vi "GVSDataView Mark Frame Below.vi"() -> ()   [LabVIEW 2013]
uses:
  <vilib>/Utility/miscctls.llb/LVPositionTypeDef.ctl
  SubVI/GVSMain Sub Window Global.vi
  GVSNew View Global.vi
panel:
  in  "sMe":string
  in  "bShow":bool=TRUE
  in  "Below":bool
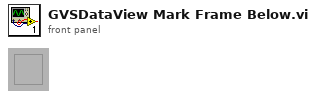
[diagram p1: front panel]
types:
  T1 = typedef "LVPositionTypeDef.ctl" = cluster{"Left":i32, "Top":i32}
  T2 = typedef "LVRectTypeDef.ctl" = cluster{"Left":i16, "Top":i16, "Right":i16, "Bottom":i16}
  T3 = typedef "Graph Main Info Cluster.ctl" = cluster{"Selected_BarIdx":i32, "Selected_PanelIdx":i32, "Graph Main VIRef":refnum<vi>, "ToolBarClick":bool, "Spliter Ref Array":refnum<vi>[], "Panel Ref Array":refnum<vi>[], "Spliter_matrix":i32[][], "Panel_matrix":i32[][], "child_spliterIdx_matrix":i32[][], "split_pos_matrix":i32[][], "Title State":bool, "sQueueName":string, "Frame nID":i32, "Graph VIRef Array":cluster{"Graph VIRef":refnum<vi>, "Panel Idx":i32, "Frame VIRef":refnum<vi>, "Icon Ring":i32, "Graph Type":string}[], "View Type":string}
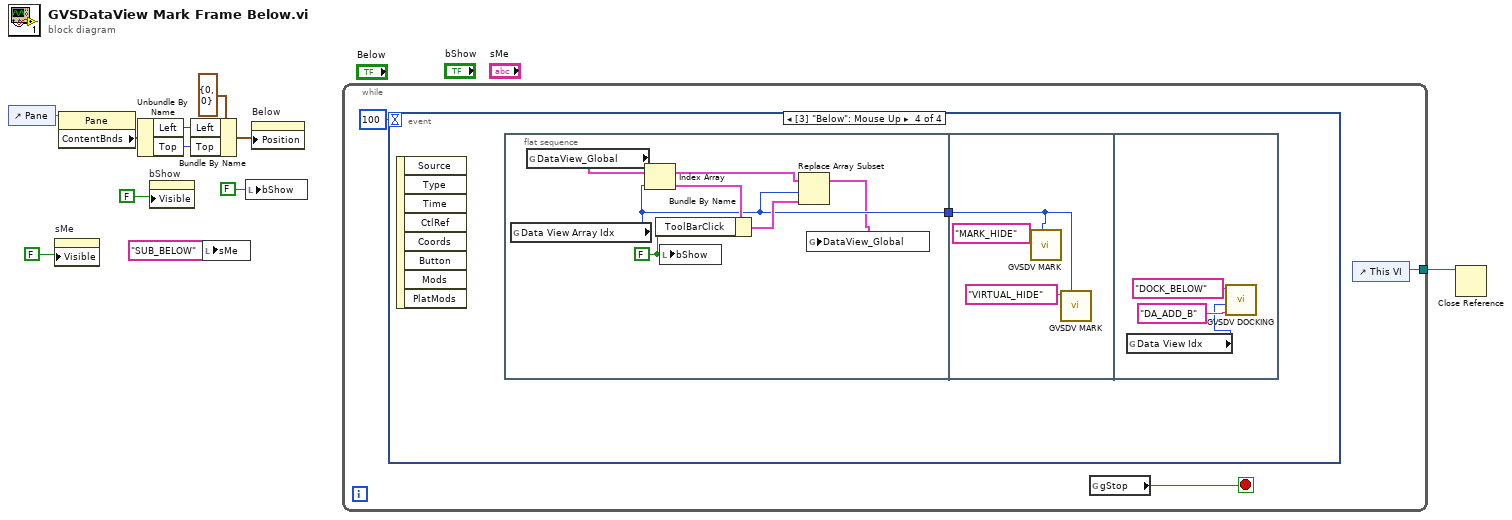
[diagram p0: block diagram]
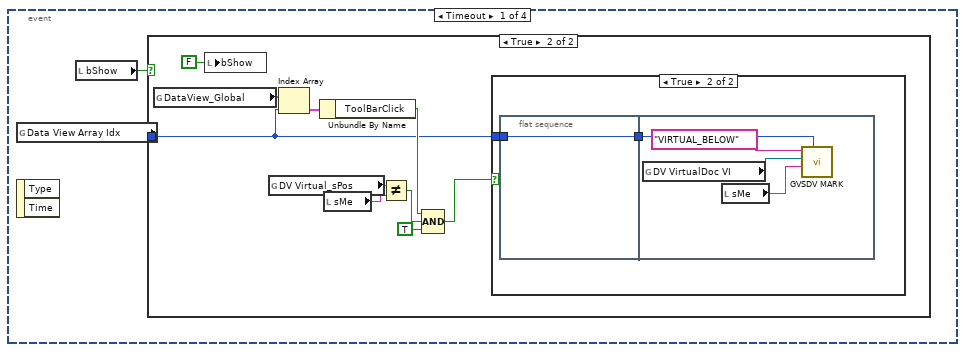
[diagram p2: hidden frame]
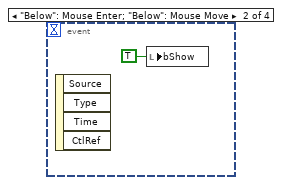
[diagram p5: hidden frame]
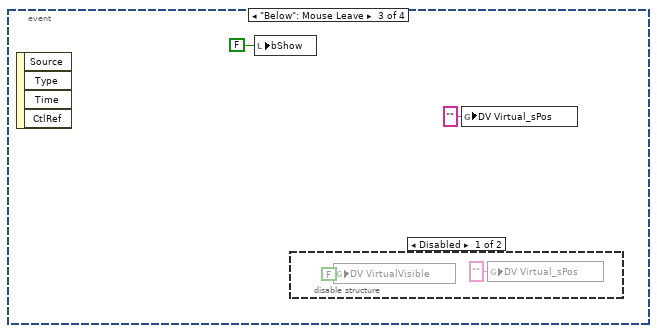
[diagram p6: hidden frame]
diagram:
  n1 = control-ref of="Pane"() -> (w11:refnum<vi>)
  n2 = property on="sMe" class="Str"("Visible"=FALSE) -> ()  [unwired: 2 in, 2 out]
  n3 = property class="Pane"(reference=w11) -> ("ContentBnds"=w10:T2)  [unwired: 1 in, 2 out]
  n4 = Unbundle By Name(w10) -> ("Left"=w9:i16, "Top"=w7:i16)
  n5 = property on="bShow" class="Bool (strict)"("Visible"=FALSE) -> ()  [unwired: 2 in, 2 out]
  n6 = Bundle By Name(cluster=T1 {"Left"=0, "Top"=0} ("Position"), "Left"=w9, "Top"=w7) -> (w6:T1)
  n7 = local write "sMe"("SUB_BELOW" ("sMe")) -> ()
  n8 = local write "bShow"(FALSE ("bShow")) -> ()
  n9 = property on="Below" class="Bool (strict)"("Position"=w6) -> ()  [unwired: 2 in, 2 out]
  n10 = while {
    tunnel: [w13] -> w1
    stop <- w12 stop-if-true
    n11 = event shown="[3] \"Below\": Mouse Up" {
      selector: _ -> [_ _ _ _]
      dyn-events: _ -> [_ _ _ _]
      timeout: 100 -> [_ _ _ _]
      event Timeout {
        n12 = global read "GVSNew View Global.vi" "Data View Array Idx"() -> (w15:i32)
        n13 = event-data() -> ()  [unwired: 3 out]
        n14 = local read "bShow"() -> (w16:bool)
        n15 = case shown="True" w16 {
          tunnel: w15 -> [_ w18]
          frame False {
          }
          frame True {
            n16 = global read "GVSNew View Global.vi" "DataView_Global"() -> (w22:T3[])
            n17 = local write "bShow"(FALSE ("bShow")) -> ()
            n18 = global read "GVSNew View Global.vi" "DV Virtual_sPos"() -> (w26:string)
            n19 = Index Array(array=w22, index=w18) -> (element=w23:T3)
            n20 = Unbundle By Name(w23) -> ("ToolBarClick"=w21:bool)
            n21 = local read "sMe"() -> (w25:string)
            n22 = Not Equal?(x=w26, y=w25) -> (x != y?=w20:bool)
            n23 = Compound Arithmetic op=AND(w21, w20, TRUE ("value")) -> (w24:bool)
            n24 = case shown="True" w24 {
              tunnel: w18 -> [_ w28]
              frame False {
              }
              frame True {
                n25 = flat-sequence {
                  tunnel: w28 -> [w29]
                  tunnel: [w29] -> w27
                  tunnel: w27 -> [w30]
                  frame #0 {
                  }
                  frame #1 {
                    n26 = global read "GVSNew View Global.vi" "DV VirtualDoc VI"() -> (w31:refnum<vi>)
                    n27 = local read "sMe"() -> (w32:string)
                    n28 = call "GVSDV MARK.vi"("sAction"="VIRTUAL_BELOW", "mVritual_VIRef"=w31, "sData"=w32, "DataView Array Index"=w30) -> ()  [unwired: 6 in, 1 out]
                  }
                }
              }
            }
          }
        }
      }
      event "Below": Mouse Enter; "Below": Mouse Move {
        n29 = event-data() -> ()  [unwired: 5 out]
        n30 = local write "bShow"(TRUE ("bShow")) -> ()
      }
      event "Below": Mouse Leave {
        n31 = event-data() -> ()  [unwired: 5 out]
        n32 = local write "bShow"(FALSE ("bShow")) -> ()
        n33 = disable-structure shown="Disabled" {
          frame Disabled {
            n34 = global write "GVSNew View Global.vi" "DV VirtualVisible"(FALSE ("VirtualVi")) -> ()
            n35 = global write "GVSNew View Global.vi" "DV Virtual_sPos"("" ("Virtual_sPos")) -> ()
          }
          frame Enabled {
          }
        }
        n36 = global write "GVSNew View Global.vi" "DV Virtual_sPos"("" ("Virtual_sPos")) -> ()
      }
      event "Below": Mouse Up {
        n37 = event-data() -> ()  [unwired: 9 out]
        n38 = flat-sequence {
          tunnel: [w41] -> w39
          tunnel: w39 -> [w47]
          frame #0 {
            w44 = FALSE ("bShow")
            n39 = global read "GVSNew View Global.vi" "Data View Array Idx"() -> (w41:i32)
            n40 = global read "GVSNew View Global.vi" "DataView_Global"() -> (w42:T3[])
            n41 = Index Array(array=w42, index=w41) -> (element=w45:T3)
            n42 = Bundle By Name(cluster=w45, "ToolBarClick"=w44) -> (w43:T3)
            n43 = local write "bShow"(w44) -> ()
            n44 = Replace Array Subset(array=w42, new element=w43, index=w41) -> (w40:T3[])
            n45 = global write "GVSNew View Global.vi" "DataView_Global"(w40) -> ()
          }
          frame #1 {
            n46 = call "GVSDV MARK.vi"("sAction"="MARK_HIDE", "DataView Array Index"=w47) -> ()  [unwired: 8 in, 1 out]
            n47 = call "GVSDV MARK.vi"("sAction"="VIRTUAL_HIDE", "DataView Array Index"=w47) -> ()  [unwired: 8 in, 1 out]
          }
          frame #2 {
            n48 = global read "GVSNew View Global.vi" "Data View Idx"() -> (w49:i32)
            n49 = call "GVSDV DOCKING.vi"("sData"="DA_ADD_B" ("Action Type"), "DataView Index"=w49, "sAction"="DOCK_BELOW") -> ()  [unwired: 5 in, 4 out]
          }
        }
      }
    }
    n50 = global read "GVSMain Sub Window Global.vi" "gStop"() -> (w12:bool)
    n51 = control-ref of="This VI"() -> (w13:refnum<vi>)
  }
  n52 = Close Reference(reference=w1) -> ()  [unwired: 1 in, 1 out]
